vi "edit io channel.vi"(6 "refresh UI":T2, 8 "error in":errorcluster, 9 "PID Loop Element":T1={"Loop ID"="", "Tags"={"Setpoint"="", "Process Variable"="", "Output"=""}, "Gains"={"P"=1.0, "I"=0.01, "D"=0.0}, "Range"={"High"=100.0, "Low"=-100.0}}, 10 "engine configuration in":refnum<class "engine configuration.lvclass">, 11 "tag bus configurable plugin module configuration in":refnum<class "Tagbus PID Module configuration.lvclass">) -> (0 "error out":errorcluster, 1 "change?":bool, 2 "engine configuration":refnum<class "engine configuration.lvclass">, 3 "tag bus configurable plugin module configuration out":refnum<class "Tagbus PID Module configuration.lvclass">)   [LabVIEW 2014, in "Tagbus PID Module editor node.lvclass"]
uses:
  Tagbus PID Module editor node.lvclass
  <vilib>/NI/Configuration Framework/Node/RefreshUIEvent.ctl
  <vilib>/NI/Module Execution Interface/Engine Configuration/engine configuration.lvclass
  module/configuration/Tagbus PID Module configuration.lvclass
  PID array element.ctl
  <vilib>/NI/Configuration Framework/serializable configuration/NISE_CEF_serializable configuration.lvclass/NISE_CEF_serializable configuration.ctl
  <vilib>/Utility/LVClass/Get LV Class Name.vi
  <vilib>/NI/Configuration Framework/error generator/NISE_error generator.vi
  <vilib>/NI/Configuration Framework/serializable configuration/NISE_CEF_serializable configuration.lvclass
  <vilib>/NI/Configuration Framework/Node/NISE_CEF_Node.lvclass
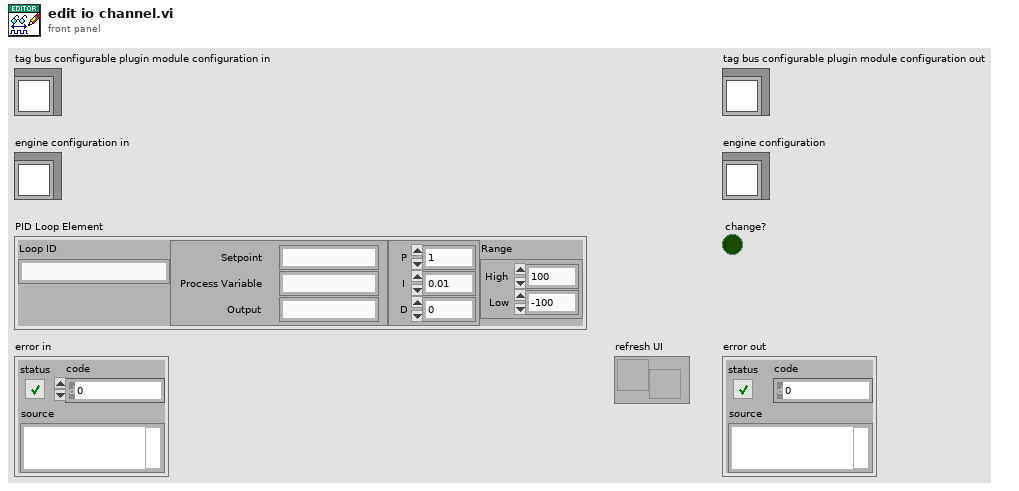
[diagram p1: front panel]
types:
  T1 = typedef "Tagbus PID Module editor node.lvclass/PID array element.ctl" = cluster{"Loop ID":string, "Tags":cluster{"Setpoint":string, "Process Variable":string, "Output":string}, "Gains":cluster{"P":dbl, "I":dbl, "D":dbl}, "Range":cluster{"High":dbl, "Low":dbl}}
  T2 = typedef "NISE_CEF_Node.lvclass/RefreshUIEvent.ctl" = refnum<user-event>
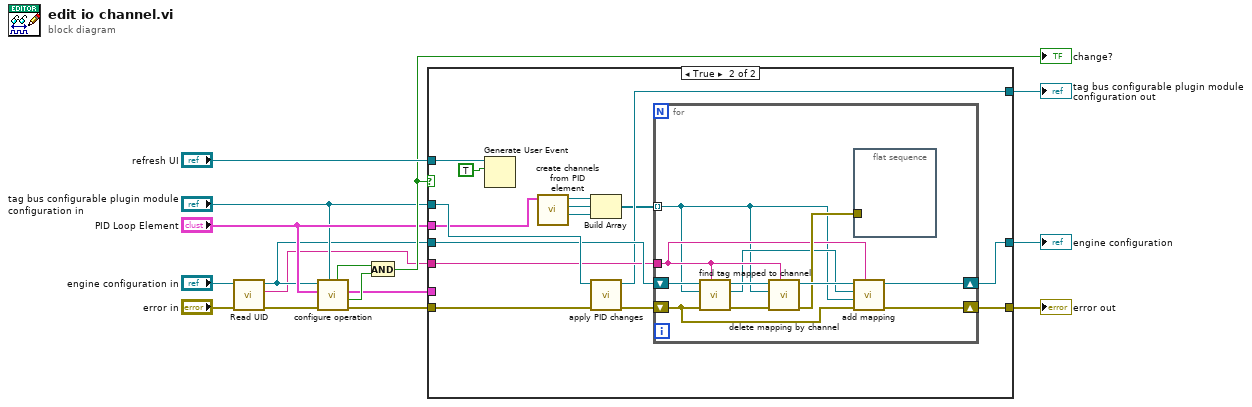
[diagram p0: block diagram]
diagram:
  n1 = call <vilib>:"Read UID.vi"("error in"="error in", "configuration in"="engine configuration in") -> ("error out"=w5:errorcluster, "instance id"=w2:string, "configuration out"=w3:refnum<class "engine configuration.lvclass">)  [unwired: 7 in]
  n2 = call "configure operation.vi"("tag bus configurable plugin module configuration"="tag bus configurable plugin module configuration in", "error in"=w5, "line item in"="PID Loop Element", "engine configuration"=w3) -> ("error out"=w9:errorcluster, "success"=w13:bool, "line item out"=w10:T1, "changed"=w12:bool)  [unwired: 4 in]
  n3 = And(x=w12, y=w13) -> (x .and. y?=w14:bool)
  "change?" <- w14
  n4 = case shown="True" w14 {
    tunnel: [w19 w27] -> w7
    tunnel: [w17 w26] -> w1
    tunnel: w3 -> [w17 w30]
    tunnel: w9 -> [w19 w33]
    tunnel: w10 -> [_ _]
    tunnel: "PID Loop Element" -> [_ w24]
    tunnel: "tag bus configurable plugin module configuration in" -> [w18 w34]
    tunnel: [w18 w25] -> w15
    tunnel: w2 -> [_ w29]
    tunnel: "refresh UI" -> [_ w32]
    frame False {
    }
    frame True {
      n5 = Generate User Event(user event=w32, event data cluster=TRUE ("event data")) -> ()  [unwired: 2 in, 2 out]
      n6 = call "create channels from PID element.vi"("line item in"=w24) -> ("channel 3"=w21:refnum<class "TBM channel.lvclass">, "channel"=w22:refnum<class "TBM channel.lvclass">, "TBM channel out"=w23:refnum<class "TBM channel.lvclass">)  [unwired: 8 in]
      n7 = Build Array(w23, w22, w21) -> (w20:refnum<class "TBM channel.lvclass">[])
      n8 = call "apply PID changes.vi"("error in"=w33, "Tagbus PID Module configuration in"=w34) -> ("error out"=w28:errorcluster, "Tagbus PID Module configuration out"=w25:refnum<class "Tagbus PID Module configuration.lvclass">)  [unwired: 8 in]
      n9 = for {
        tunnel: w29 -> [w39]
        shift-right: [w44] -> w27
        shift-left: w28 -> [w37]
        shift-right: [w43] -> w26
        shift-left: w30 -> [w41]
        tunnel: w20 -> [w35] mode=indexing
        n10 = call <vilib>:"find tag mapped to channel.vi"("owner"=w39, "error in"=w37, "channel"=w35, "engine configuration in"=w41) -> ("error out"=w38:errorcluster, "tag"=w36:refnum<class "tag descriptor.lvclass">, "engine configuration out"=w40:refnum<class "engine configuration.lvclass">)  [unwired: 5 in]
        n11 = call <vilib>:"delete mapping by channel.vi"("owner ID"=w39, "error in"=w38, "channel"=w35, "engine configuration in"=w40) -> ("error out"=w42:errorcluster, "engine configuration out"=w45:refnum<class "engine configuration.lvclass">)  [unwired: 6 in]
        n12 = flat-sequence {
          tunnel: w42 -> [_]
          frame #0 {
          }
        }
        n13 = call <vilib>:"add mapping.vi"("owner ID"=w39, "error in"=w37, "channel"=w35, "tag descriptor"=w36, "engine configuration"=w45) -> ("error out"=w44:errorcluster, "engine configuration out"=w43:refnum<class "engine configuration.lvclass">)  [unwired: 5 in]
      }
    }
  }
  "engine configuration" <- w1
  "tag bus configurable plugin module configuration out" <- w15
  "error out" <- w7
